vi "Build OAuth Handle.vi"(5 "Version (1.0)":string="1.0", 7 "Signature Method (HMAC-SHA1)":T1=enum."HMAC-SHA1", 8 "Access Secret":string, 9 "Access Token":string, 10 "Client Secret":string, 11 "Client Token":string) -> (3 "OAuth Handle":T2={"Signature Method"=enum."HMAC-SHA1", "Version"="1.0", "Client"={"Token"="", "Secret"=""}, "Access"={"Token"="", "Secret"=""}})   [LabVIEW 2011, in "i3-oauth.lvlib"]
uses:
  i3-oauth.lvlib
  Controls/OAuth Handle.ctl
  Controls/Signature Method.ctl
  Controls/Credentials.ctl
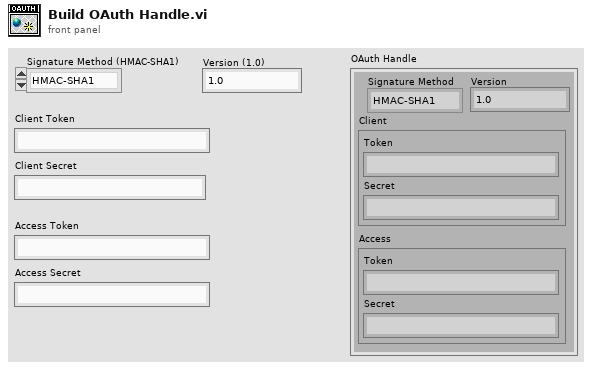
[diagram p1: front panel]
types:
  T1 = typedef "i3-oauth.lvlib/Signature Method.ctl" = enum16{"HMAC-MD5", "HMAC-SHA1", "HMAC-SHA224", "HMAC-SHA256", "HMAC-SHA384", "HMAC-SHA512"}
  T2 = typedef "i3-oauth.lvlib/OAuth Handle.ctl" = cluster{"Signature Method":T1, "Version":string, "Client":T3, "Access":T3}
  T3 = typedef "i3-oauth.lvlib/Credentials.ctl" = cluster{"Token":string, "Secret":string}
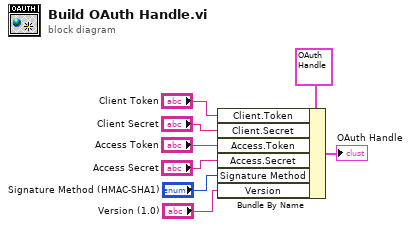
[diagram p0: block diagram]
diagram:
  n1 = Bundle By Name(cluster=T2 {"Signature Method"=enum."HMAC-SHA1", "Version"="1.0", "Client"={"Token"="", "Secret"=""}, "Access"={"Token"="", "Secret"=""}} ("OAuth Handle"), "Client.Token"="Client Token", "Client.Secret"="Client Secret", "Access.Token"="Access Token", "Access.Secret"="Access Secret", "Signature Method"="Signature Method (HMAC-SHA1)", "Version"="Version (1.0)") -> (→"OAuth Handle":T2)
